vi "initialize.vi"(0 "HGV_PVBase":refnum<class "HGF_PVBase.lvclass">, 3 "initializationData":variant, 5 "error in (no error)":errorcluster, 7 "binaryString":string, 8 "I8 Array":i8[](array[numeric]), 9 "prependSize? (T)":bool, 11 "byteOrder (0:big-endian, network order)":T1(ring)) -> (14 "HGV_PVBase":refnum<class "HGF_PVBase.lvclass">, 17 "found?":bool, 19 "error out":errorcluster)   [LabVIEW 2014, in "HGF_BaseClasses.lvlib" / "HGF_PVBase.lvclass"]
doc: "This is a dynamic dispatch VI to be implemented by child classes to initialize their attributes.\n\n<B>Recommendation:</B> Use Variant for initialization data."
uses:
  HGF_PVBase.lvclass
  HGF_PVDataConverter/HGF_PVDataConverter.lvclass
  HGF_Base/HGF_Base.lvclass
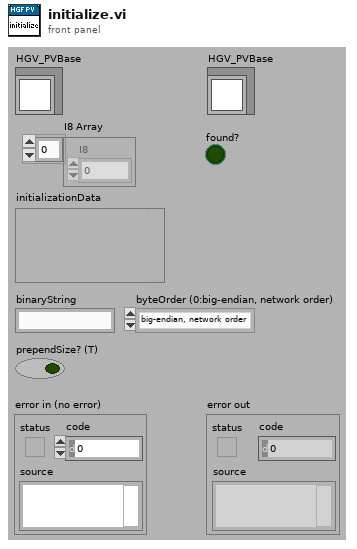
[diagram p1: front panel]
types:
  T1 = enum16{"big-endian, network order", "native, host order", "little-endian"}
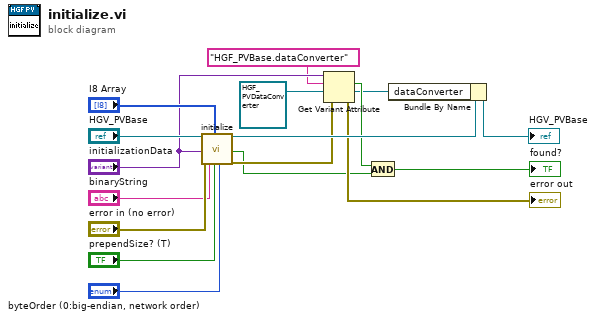
[diagram p0: block diagram]
diagram:
  n1 = call-parent "initialize.vi"("HGF_Base"="HGV_PVBase", "initializationData"="initializationData", "error in (no error)"="error in (no error)", "binaryString"="binaryString", "I8 Array"="I8 Array", "prependSize? (T)"="prependSize? (T)", "byteOrder (0:big-endian, network order)"="byteOrder (0:big-endian, network order)") -> ("dup HGF_Base"=w14:refnum<class "HGF_PVBase.lvclass">, "found?"=w9:bool, "error out"=w11:errorcluster)  [unwired: 1 in, 9 out]
  n2 = Get Variant Attribute(Variant="initializationData", name="HGF_PVBase.dataConverter", default value (empty Variant)=refnum<class "HGF_PVDataConverter.lvclass"> refnum ("HGF_BaseClasses.lvlib:HGF_PVDataConverter.lvclass"), error in=w11) -> (found=w2:bool, value=w1:refnum<class "HGF_PVDataConverter.lvclass">, error out=→"error out":errorcluster)  [unwired: 1 out]
  n3 = And(x=w2, y=w9) -> (x .and. y?=→"found?":bool)
  n4 = Bundle By Name(cluster=w14, "dataConverter"=w1) -> (→"HGV_PVBase":refnum<class "HGF_PVBase.lvclass">)
